vi "TW Substitute the assigned name for Interactive Test.vi"(8 "error in":errorcluster, 10 "Project Name":string, 11 "Name to VI Map":map{string, refnum<vi>}(c390)) -> (0 "error out":errorcluster)   [LabVIEW 2021, in "Plugin Generator.lvlib"]
uses:
  Plugin Generator.lvlib
  <vilib>/Utility/traverseref.llb/TRef TravTarget.ctl
  <vilib>/Utility/traverseref.llb/VI Scripting - Traverse.lvlib
panel:
  out "Array":string[](array[string])
  in  "vi path":path
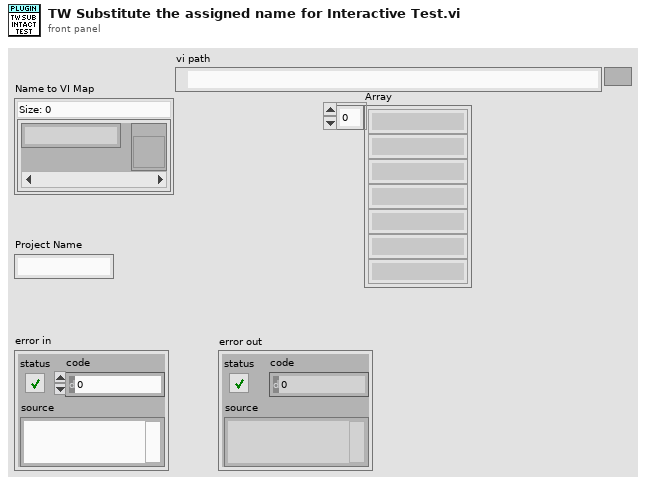
[diagram p1: front panel]
types:
  T1 = typedef "TRef TravTarget.ctl" = enum16{"FP", "BD", "Other"}
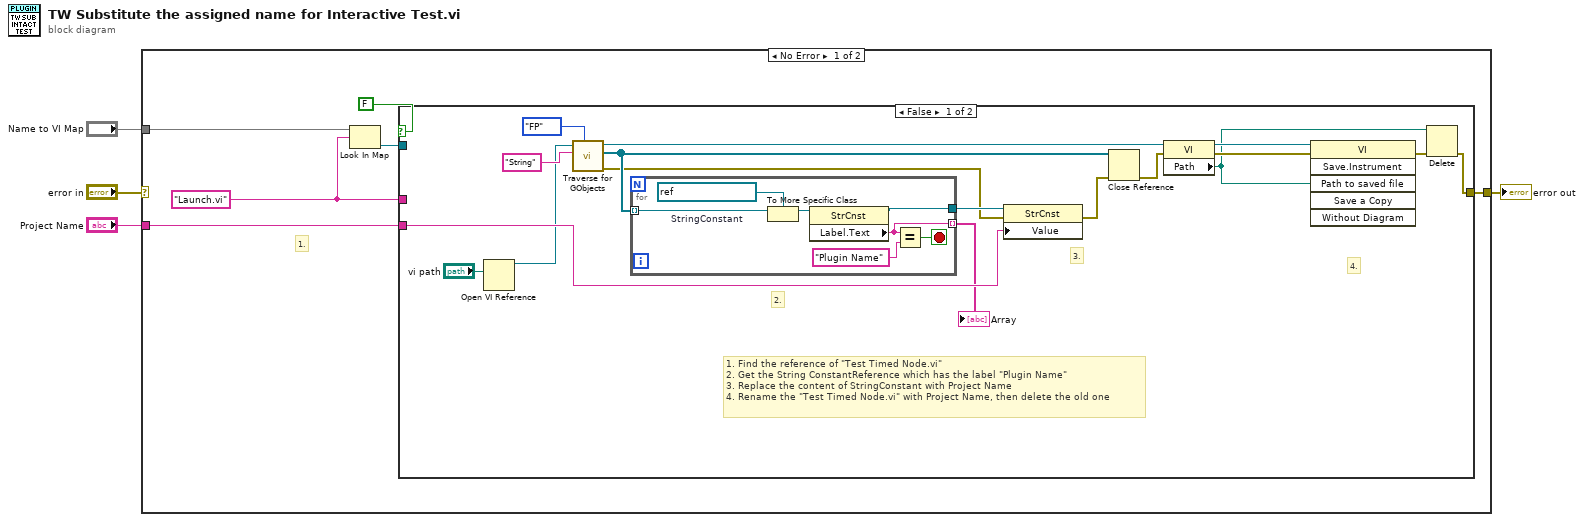
[diagram p0: block diagram]
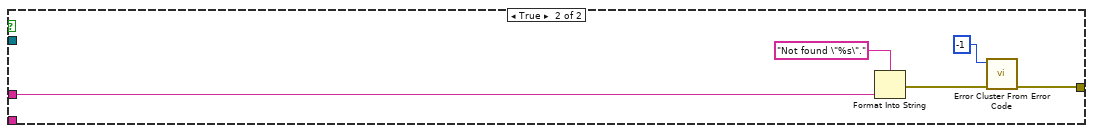
[diagram p2: hidden frame]
diagram:
  n1 = case shown="No Error" "error in" {
    selector: "error in" -> [_ w40]
    tunnel: [w10 w40] -> w4
    tunnel: "Project Name" -> [w9 _]
    tunnel: "Name to VI Map" -> [w8 _]
    frame No Error {
      w6 = "Launch.vi" ("String")
      # "1."
      n2 = Look In Map(map=w8, key=w6) -> (value=w7:refnum<vi>)  [unwired: 1 in, 1 out]
      n3 = case shown="False" FALSE {
        tunnel: [w27 w39] -> w10
        tunnel: w9 -> [w15 _]
        tunnel: w7 -> [_ _]
        tunnel: w6 -> [_ w35]
        frame False {
          # "4."
          # "3."
          # "2."
          # "1. Find the reference of \"Test Timed Node.vi\"\n2. Get the String ConstantReference which has the label \"Plugin Name\"\n3. Replace the content of StringConstant with Project Name\n4. Rename the \"Test Timed Node.vi\" with Project Name, then delete the old one"
          n4 = Open VI Reference(vi path="vi path") -> (vi reference=w13:refnum<vi>)  [unwired: 5 in, 1 out]
          n5 = call <vilib>:"Traverse for GObjects.vi"("Traverse Target"=TRef_TravTarget."FP", "Class Name"="String", "VI Refnum"=w13) -> ("error out"=w17:errorcluster, "References"=w22:refnum<vi>[], "dup VI Refnum"=w18:refnum<vi>)  [unwired: 5 in, 1 out]
          n6 = for {
            tunnel: w22 -> [w34] mode=indexing
            tunnel: [w29] -> w21
            tunnel: [w28] -> w11 mode=indexing
            stop <- w30 stop-if-true
            w33 = refnum<vi> refnum  # StringConstant
            n7 = To More Specific Class(target class=w33, reference=w34) -> (specific class reference=w32:refnum<vi>)  [unwired: 1 in, 1 out]
            n8 = property class="StrCnst"(reference=w32) -> (reference out=w29:refnum<vi>, "Label.Text"=w28:string)  [unwired: 1 in, 1 out]
            n9 = Equal?(x=w28, y="Plugin Name") -> (x = y?=w30:bool)
          }
          "Array" <- w11
          n10 = property class="StrCnst"(reference=w21, error in=w17, "Value"=w15) -> (error out=w23:errorcluster)  [unwired: 1 out]
          n11 = Close Reference(reference=w22, error in (no error)=w23) -> (error out=w16:errorcluster)
          n12 = property class="VI"(reference=w18, error in=w16) -> (reference out=w26:refnum<vi>, error out=w25:errorcluster, "Path"=w14:path)
          n13 = invoke class="VI" method="Save.Instrument"(reference=w26, error in=w25, "Path to saved file"=w14) -> (error out=w24:errorcluster)  [unwired: 3 in, 5 out]
          n14 = Delete(path (use dialog)=w14, error in=w24) -> (error out=w27:errorcluster)  [unwired: 3 in, 2 out]
        }
        frame True {
          n15 = Format Into String(format string="Not found \"%s\"." ("error message (\"\")"), w35) -> (error out=w37:errorcluster)  [unwired: 2 in, 1 out]
          n16 = call <vilib>:"Error Cluster From Error Code.vi"("error in (no error)"=w37, "error code (0)"=-1) -> ("error out"=w39:errorcluster)  [unwired: 7 in]
        }
      }
    }
    frame Error {
    }
  }
  "error out" <- w4
